vi "Get UDP Buffer Size.vi"(9 "Decimation":i32, 10 "History Length":dbl, 11 "Root":refnum<k24>) -> (3 "Buffer Size":i32)   [LabVIEW 2013, in "Workspace MultiY Graph.lvlib"]
uses:
  Workspace MultiY Graph.lvlib
  NationalInstruments.VeriStand.SystemStorage
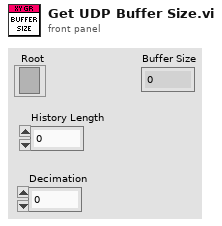
[diagram p1: front panel]
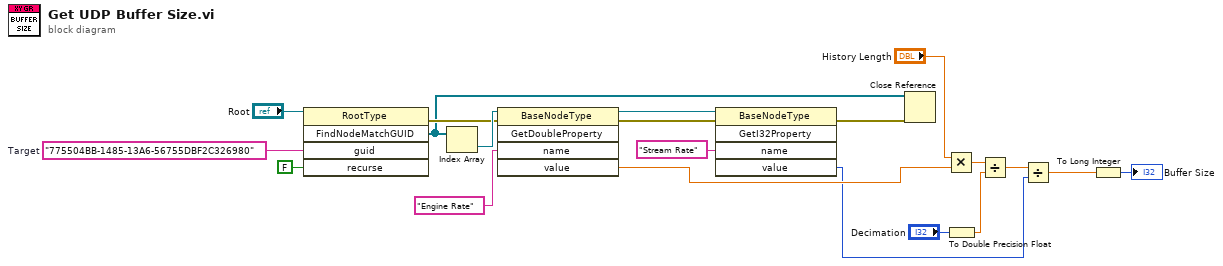
[diagram p0: block diagram]
diagram:
  w14 = "775504BB-1485-13A6-56755DBF2C326980"  # Target
  n1 = invoke class="RootType" method="FindNodeMatchGUID"(reference="Root", "guid"=w14, "recurse"=FALSE) -> (error out=w10:errorcluster, "FindNodeMatchGUID"=w8:refnum<k24>[])  [unwired: 2 in, 3 out]
  n2 = Index Array(array=w8) -> (element=w12:refnum<k24>)  [unwired: 1 in]
  n3 = invoke class="BaseNodeType" method="GetDoubleProperty"(reference=w12, error in=w10, "name"="Engine Rate") -> (reference out=w6:refnum<k24>, error out=w7:errorcluster, "value"=w9:dbl)  [unwired: 2 in, 2 out]
  n4 = invoke class="BaseNodeType" method="GetI32Property"(reference=w6, error in=w7, "name"="Stream Rate") -> (error out=w5:errorcluster, "value"=w2:i32)  [unwired: 2 in, 3 out]
  n5 = Close Reference(reference=w8, error in (no error)=w5) -> ()  [unwired: 1 out]
  n6 = Multiply(x="History Length", y=w9) -> (x*y=w18:dbl)
  n7 = To Double Precision Float(number="Decimation") -> (double precision float=w16:dbl)
  n8 = Divide(x=w18, y=w16) -> (x/y=w3:dbl)
  n9 = Divide(x=w3, y=w2) -> (x/y=w1:dbl)
  n10 = To Long Integer(number=w1) -> (32bit integer=→"Buffer Size":i32)
